vi "instructions.vi"(8 "error in (no error)":errorcluster, 11 "simonMessages in":refnum<class "simonMessages.lvclass">) -> (0 "error out":errorcluster, 3 "simonMessages out":refnum<class "simonMessages.lvclass">)   [LabVIEW 2019, in "simonMessages.lvclass"]
uses:
  simonMessages.lvclass
  simonMessages.lvclass/simonMessages.ctl
  TextDisplay/TextDisplay Class.lvclass
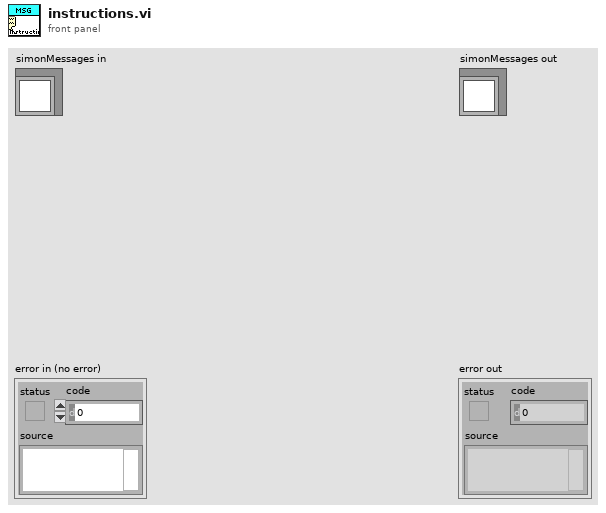
[diagram p1: front panel]
types:
  T1 = cluster{"Text":string, "Size":u8, "Justification":enum16{"Left", "Center", "Right"}, "Display Type":string}
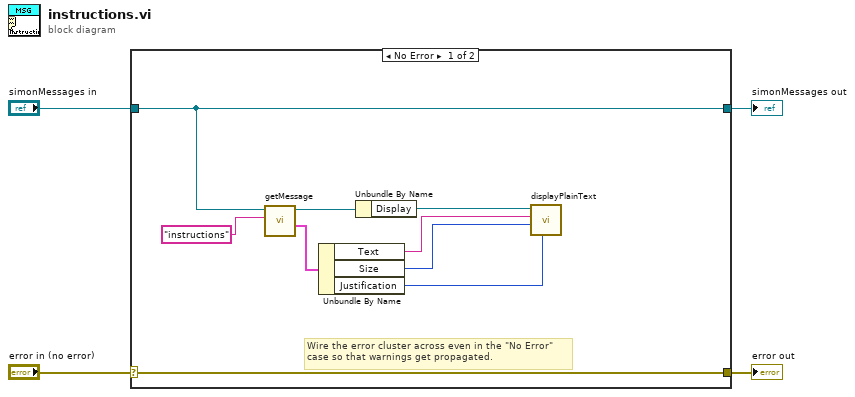
[diagram p0: block diagram]
diagram:
  n1 = case shown="No Error" "error in (no error)" {
    selector: "error in (no error)" -> [w13 w15]
    tunnel: [w13 w15] -> w3
    tunnel: [w9 w14] -> w1
    tunnel: "simonMessages in" -> [w9 w14]
    frame No Error {
      # "Wire the error cluster across even in the \"No Error\"\ncase so that warnings get propagated."
      n2 = call "getMessage.vi"("key"="instructions", "simonMessages in"=w9) -> ("Message Cluster"=w8:T1, "simonMessages out"=w11:refnum<class "simonMessages.lvclass">)  [unwired: 7 in, 1 out]
      n3 = Unbundle By Name(w8) -> ("Text"=w7:string, "Size"=w6:u8, "Justification"=w5:enum16{"Left", "Center", "Right"})
      n4 = Unbundle By Name(w11) -> ("Display"=w12:refnum<class "TextDisplay Class.lvclass">)
      n5 = call "displayPlainText.vi"("Justification"=w5, "Font Size"=w6, "Text In"=w7, "TextDisplay Class in"=w12) -> ()  [unwired: 6 in, 2 out]
    }
    frame Error {
    }
  }
  "error out" <- w3
  "simonMessages out" <- w1
